vi "HandleVersionMutation.vi"(4 "To Version":u16, 6 "From Version":u16, 8 "error in (no error)":errorcluster, 10 "SerializableData in":variant, 11 "Bill Murray":refnum<class "Bill Murray.lvclass">) -> (0 "error out":errorcluster, 2 "SerializableData out":variant, 3 "Bill Murray":refnum<class "Bill Murray.lvclass">)   [LabVIEW 2020, in "Bill Murray.lvclass"]
uses:
  Bill Murray.lvclass
  SerializableData_v1.ctl
  Golf Club.lvclass
  <vilib>/Utility/error.llb/Error Cluster From Error Code.vi
  <vilib>/ErrorRing/Error Ring.xnode
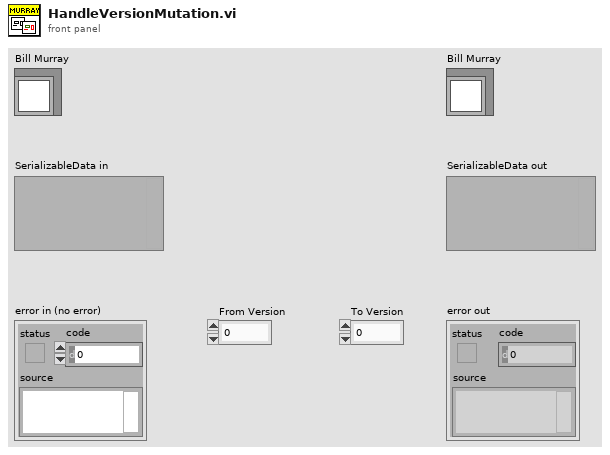
[diagram p1: front panel]
types:
  T1 = typedef "Bill Murray.lvclass/SerializableData_v1.ctl" = cluster{"Nickname":string, "Golf Club":refnum<class "Golf Club.lvclass">}
  T2 = typedef "Bill Murray.lvclass/SerializableData.ctl" = cluster{"Golf Club":refnum<class "Golf Club.lvclass">, "Nicknames":string[]}
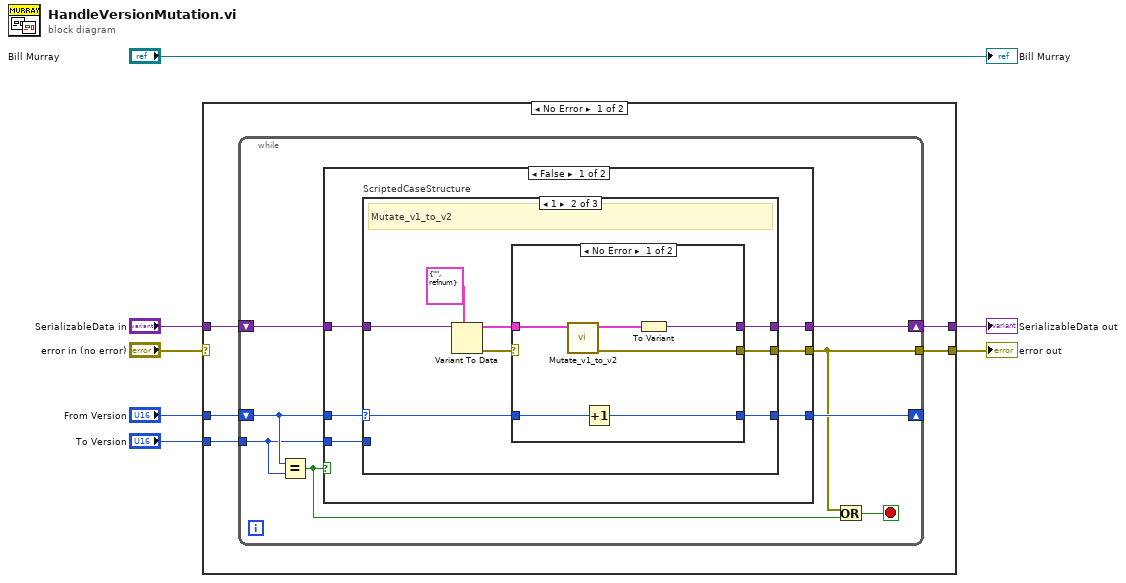
[diagram p0: block diagram]
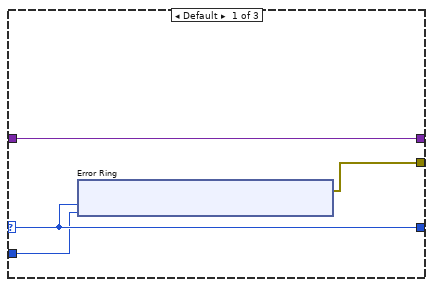
[diagram p2: hidden frame]
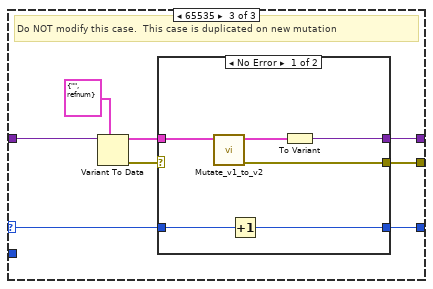
[diagram p4: hidden frame]
diagram:
  n1 = case shown="No Error" "error in (no error)" {
    selector: "error in (no error)" -> [_ w74]
    tunnel: "From Version" -> [w12 _]
    tunnel: "To Version" -> [w11 _]
    tunnel: "SerializableData in" -> [w10 w73]
    tunnel: [w9 w74] -> w4
    tunnel: [w8 w73] -> w3
    frame No Error {
      n2 = while {
        tunnel: w11 -> [w13]
        shift-right: [w17] -> _
        shift-left: w12 -> [w20]
        shift-right: [w18] -> w8
        shift-left: w10 -> [w19]
        tunnel: [w14] -> w9
        stop <- w15 stop-if-true
        n3 = Equal?(x=w20, y=w13) -> (x = y?=w16:bool)
        n4 = case shown="False" w16 {
          tunnel: w20 -> [w26 w72]
          tunnel: w19 -> [w25 w71]
          tunnel: [w24 w71] -> w18
          tunnel: [w23 _] -> w14
          tunnel: [w22 w72] -> w17
          tunnel: w13 -> [w21 _]
          frame False {
            n5 = case "ScriptedCaseStructure" shown="1" w26 {
              selector: w26 -> [w30 w40 w56]
              tunnel: w25 -> [w28 w46 w62]
              tunnel: [w28 w43 w59] -> w24
              tunnel: [w29 w42 w58] -> w23
              tunnel: [w30 w41 w57] -> w22
              tunnel: w21 -> [w27 _ _]
              frame Default {
                n6 = xnode "Error Ring"("parameter 0"=w30, "parameter 1"=w27) -> ("error out"=w29:errorcluster)
              }
              frame 1 {
                # "Mutate_v1_to_v2"
                n7 = Variant To Data(type=T1 {"Nickname"="", "Golf Club"=refnum} ("SerializableData"), Variant=w46) -> (data=w44:T1, error out=w45:errorcluster)  [unwired: 1 in]
                n8 = case shown="No Error" w45 {
                  selector: w45 -> [_ w54]
                  tunnel: w44 -> [w49 _]
                  tunnel: [w52 _] -> w43
                  tunnel: [w47 w54] -> w42
                  tunnel: w40 -> [w51 w53]
                  tunnel: [w50 w53] -> w41
                  frame No Error {
                    n9 = call "Mutate_v1_to_v2.vi"("SerializableData_v1"=w49) -> ("error out"=w47:errorcluster, "SerializableData"=w48:T2)  [unwired: 9 in]
                    n10 = Increment(x=w51) -> (x+1=w50:u16)
                    n11 = To Variant(anything=w48) -> (Variant=w52:variant)
                  }
                  frame Error {
                  }
                }
              }
              frame 65535 {
                # "Do NOT modify this case.  This case is duplicated on new mutation"
                n12 = Variant To Data(type=T1 {"Nickname"="", "Golf Club"=refnum} ("SerializableData"), Variant=w62) -> (data=w60:T1, error out=w61:errorcluster)  [unwired: 1 in]
                n13 = case shown="No Error" w61 {
                  selector: w61 -> [_ w70]
                  tunnel: w60 -> [w65 _]
                  tunnel: [w68 _] -> w59
                  tunnel: [w63 w70] -> w58
                  tunnel: w56 -> [w67 w69]
                  tunnel: [w66 w69] -> w57
                  frame No Error {
                    n14 = call "Mutate_v1_to_v2.vi"("SerializableData_v1"=w65) -> ("error out"=w63:errorcluster, "SerializableData"=w64:T2)  [unwired: 9 in]
                    n15 = Increment(x=w67) -> (x+1=w66:u16)
                    n16 = To Variant(anything=w64) -> (Variant=w68:variant)
                  }
                  frame Error {
                  }
                }
              }
            }
          }
          frame True {
          }
        }
        n17 = Or(x=w14, y=w16) -> (x .or. y?=w15:bool)
      }
    }
    frame Error {
    }
  }
  "error out" <- w4
  "SerializableData out" <- w3
  "Bill Murray" <- "Bill Murray"
